vi "Show where code is waiting.vi"(1 "Loop index":i32, 2 "Wait (ms)":u32, 3 "Message":string) -> ()   [LabVIEW 2020]
panel:
  in  "Button":bool=TRUE
  out "Message Display":string
  out "Last Written to:":string
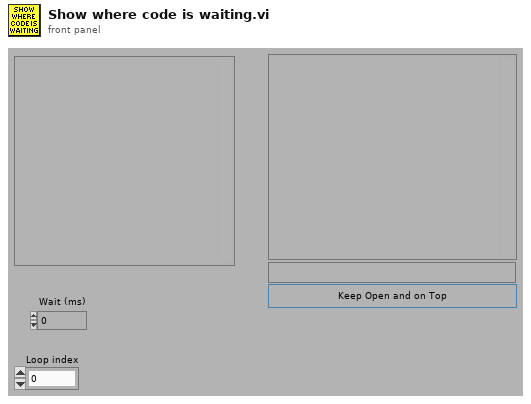
[diagram p1: front panel]
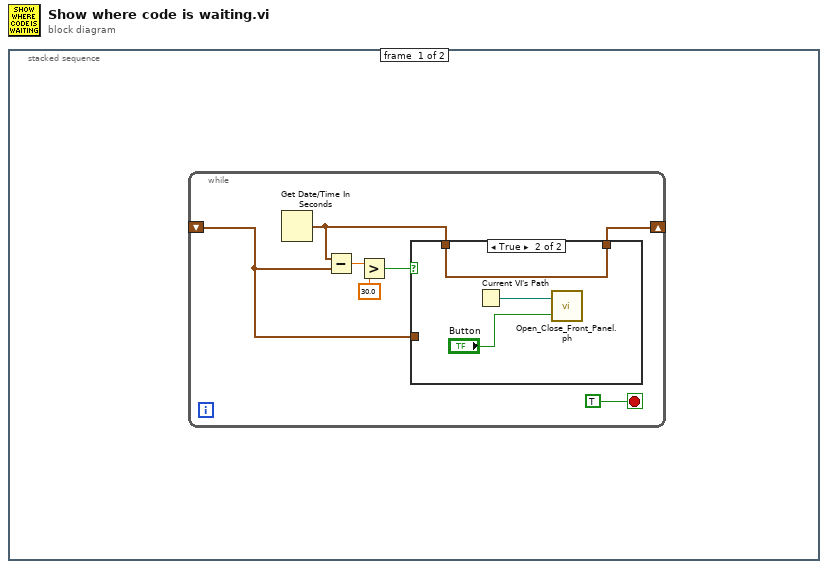
[diagram p0: block diagram]
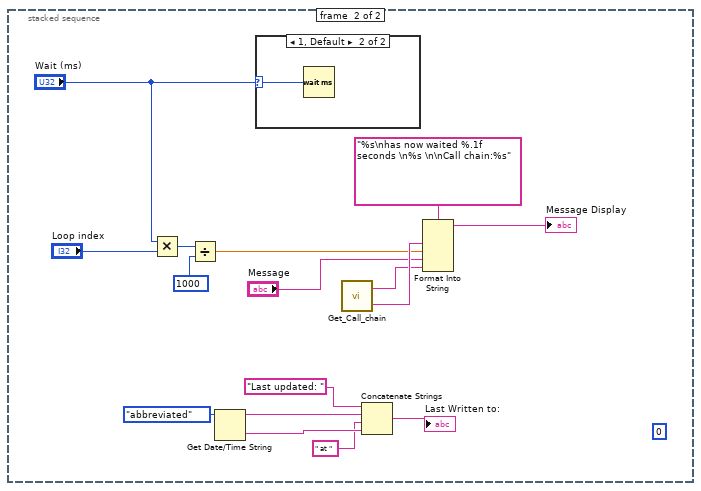
[diagram p3: hidden frame]
diagram:
  n1 = stacked-sequence {
    frame #0 {
      n2 = while {
        shift-right: [w3] -> _
        shift-left: _ -> [w1]
        stop <- TRUE stop-if-true
        n3 = Get Date/Time In Seconds() -> (seconds since 1Jan1904=w2:timestamp)
        n4 = Subtract(x=w2, y=w1) -> (x-y=w7:dbl)
        n5 = Greater?(x=w7, y=30.0) -> (0:w4:bool)
        n6 = case shown="True" w4 {
          tunnel: [w8 w11] -> w3
          tunnel: w2 -> [_ w11]
          tunnel: w1 -> [w8 _]
          frame False {
          }
          frame True {
            n7 = Current VI's Path() -> (path=w10:path)
            n8 = call "Open_Close_Front_Panel.ph.vi"("openWindow (T)"="Button", "VI path"=w10) -> ()  [unwired: 1 in, 1 out]
          }
        }
      }
    }
    frame #1 {
      (unwired) 0
      n9 = Multiply(x="Wait (ms)", y="Loop index") -> (x*y=w22:u32)
      n10 = Divide(x=w22, y=1000) -> (x/y=w17:dbl)
      n11 = Get Date/Time String(date format (0)=enum16{"short", "long", "abbreviated"}."abbreviated") -> (date string=w27:string, time string=w26:string)  [unwired: 2 out]
      n12 = case shown="1, Default" "Wait (ms)" {
        selector: "Wait (ms)" -> [_ w28]
        frame 0 {
        }
        frame 1, Default {
          n13 = Wait (ms)(milliseconds to wait=w28) -> ()  [unwired: 1 out]
        }
      }
      n14 = call "Get_Call_chain.vi"() -> ("Output String"=w15:string, "VI to open"=w18:string)  [unwired: 1 in]
      n15 = Concatenate Strings("Last updated: ", w27, " at ", w26) -> (→"Last Written to:":string)
      n16 = Format Into String(format string="%s\nhas now waited %.1f seconds \n%s \n\nCall chain:%s", w18, w17, "Message", w15) -> (resulting string=→"Message Display":string)  [unwired: 2 in, 1 out]
    }
  }
